vi "Close Port.vi"(8 "error in (no error)":errorcluster, 11 "Serial Base in":refnum<class "Serial Base.lvclass">) -> (0 "error out":errorcluster, 3 "Serial Base out":refnum<class "Serial Base.lvclass">)   [LabVIEW 2022 SP3, in "Serial Base.lvclass"]
uses:
  Serial Base.lvclass
  Object Argument--cluster.ctl
  Termination Character--enum.ctl
  Data Argument--cluster.ctl
  Serial Base.lvclass/Serial Base.ctl
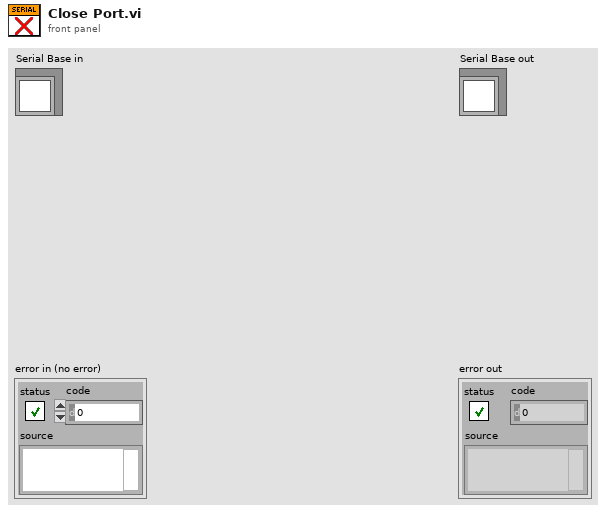
[diagram p1: front panel]
types:
  T1 = typedef "Serial Base.lvclass/Data Argument--cluster.ctl" = cluster{"Status":string}
  T2 = typedef "Serial Base.lvclass/Object Argument--cluster.ctl" = cluster{"Com Port":refnum<visa-resource-name>, "baud rate":u32, "data bits":u16, "Termination Char":T3, "parity":enum16{"None", "Odd", "Even", "Mark", "Space"}, "stop bits":u16, "flow control ":u16, "timeout ":u32}
  T3 = typedef "Serial Base.lvclass/Termination Character--enum.ctl" = enum16{"none", "\\r\\n", "\\r", "\\n"}
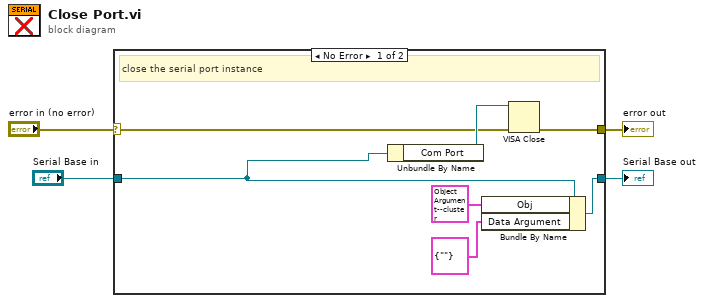
[diagram p0: block diagram]
diagram:
  n1 = case shown="No Error" "error in (no error)" {
    selector: "error in (no error)" -> [w10 w13]
    tunnel: [w9 w13] -> w3
    tunnel: [w7 w12] -> w1
    tunnel: "Serial Base in" -> [w8 w12]
    frame No Error {
      # "close the serial port instance"
      n2 = Unbundle By Name(w8) -> ("Com Port"=w11:refnum<visa-resource-name>)
      n3 = Bundle By Name(cluster=w8, "Obj"=T2 {"Com Port"="", "baud rate"=0, "data bits"=8, "Termination Char"=enum."\\r\\n", "parity"=enum."None", "stop bits"=0, "flow control "=0, "timeout "=10000}, "Data Argument"=T1 {"Status"=""}) -> (w7:refnum<class "Serial Base.lvclass">)
      n4 = VISA Close(VISA resource name=w11, error in (no error)=w10) -> (error out=w9:errorcluster)
    }
    frame Error {
    }
  }
  "error out" <- w3
  "Serial Base out" <- w1
